vi "Capacitance Bridge.vi"(1 "Action":T4=enum."Identify", 2 "Parameters":variant) -> (6 "Output":variant, 7 "Stop":bool)   [LabVIEW 2020]
uses:
  Sub Controls/Instrument Actions.ctl
  Sub Controls/Public.ctl
  Sub Controls/Instrument Match.ctl
  Sub Controls/Factory Reset.ctl
  Sub Controls/Scan Output.ctl
  Sub Controls/Instrument IDN.ctl
  Sub Controls/User Event Command.ctl
panel:
  out "Firmware Warning":string="\nUPDATE Firmware!\nVersion must be ≥ AH2X0428"
  in  "Factory Reset":T1
  out "Average Time (mS)":u32
  in  "Read Frequency":bool
  out "Is AH2500?":bool
  out "Title":string="Capacitance Bridge"
  out "Frequency":dbl
  in  "Average Time":u32(slide)=4 max=15 step=1 scale=0.0..1.0
  in  "Return Dissapation":u8(slide) max=5 step=1 scale=0.0..5.0
  in  "VISA resource name":refnum<visa-resource-name>
  in  "Instruments":T2[](array[typedef])=[{"Model"="2500A", "Manufacturer"="ANDEEN-HAGERLING", "Term Character"="", "Wait Time (mS)"=0, "Wait for SRQ"=FALSE, "Type"="Capacitance Bridge"}, {"Model"="AH2700A", "Manufacturer"="ANDEEN-HAGERLING", "Term Character"="", "Wait Time (mS)"=0, "Wait for SRQ"=FALSE, "Type"="Capacitance Bridge"}]
  out "Model":string
  in  "Address":u16(ring)
  in  "Public":T3
  out "Measurement":dbl[](array[numeric]) format="%^.2e"
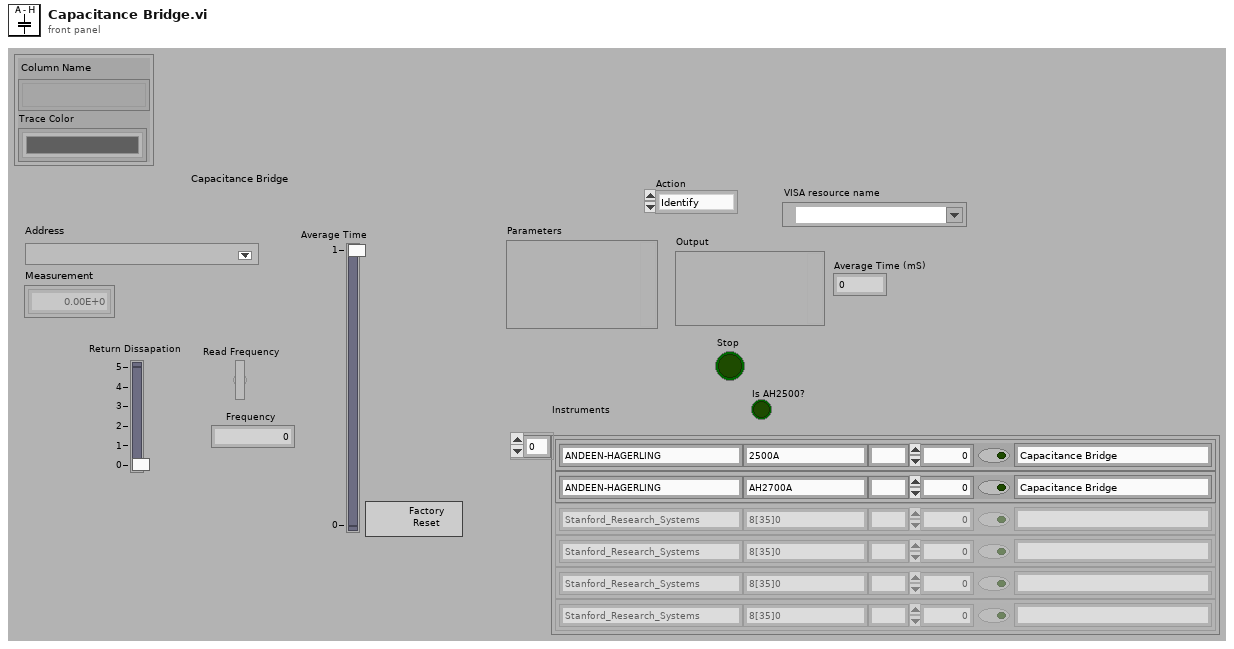
[diagram p1: front panel]
types:
  T1 = typedef "Factory Reset.ctl" = bool
  T2 = typedef "Instrument Match.ctl" = cluster{"Model":string, "Manufacturer":string, "Term Character":string, "Wait Time (mS)":u32, "Wait for SRQ":bool, "Type":string}
  T3 = typedef "Public.ctl" = cluster{"Column Name":string[], "Trace Color":u32[]}
  T4 = typedef "Instrument Actions.ctl" = enum16{"Scan", "Identify", "New", "Configure", "Initialize", "Test", "Read", "Close"}
  T5 = typedef "Scan Output.ctl" = cluster{"Manufacturer":string, "Model":string, "Info":string, "Revision":string, "error out":errorcluster}
  T6 = typedef "Instrument IDN.ctl" = cluster{"VISA Address":string, "Status":u16, "Manufacturer":string, "Model":string, "Info":string, "Info 2":string, "Misc Data":variant}
  T7 = typedef "User Event Command.ctl" = enum32{"Stop Config"}
  T8 = cluster{"VISA resource name":refnum<visa-resource-name>, string}
  T9 = typedef "Instrument Properties.ctl" = cluster{"Public":T3, "Private":T10}
  T10 = typedef "Private.ctl" = cluster{"Path":path, "VI Refnum":T11, "Name":string, "# of Values":i32, "Scale Factors":dbl[], "Display":T12[], "Offset":dbl[]}
  T11 = typedef "Instrument Ref.ctl" = refnum<vi>
  T12 = typedef "SystemCheckBox-resize.ctl" = bool
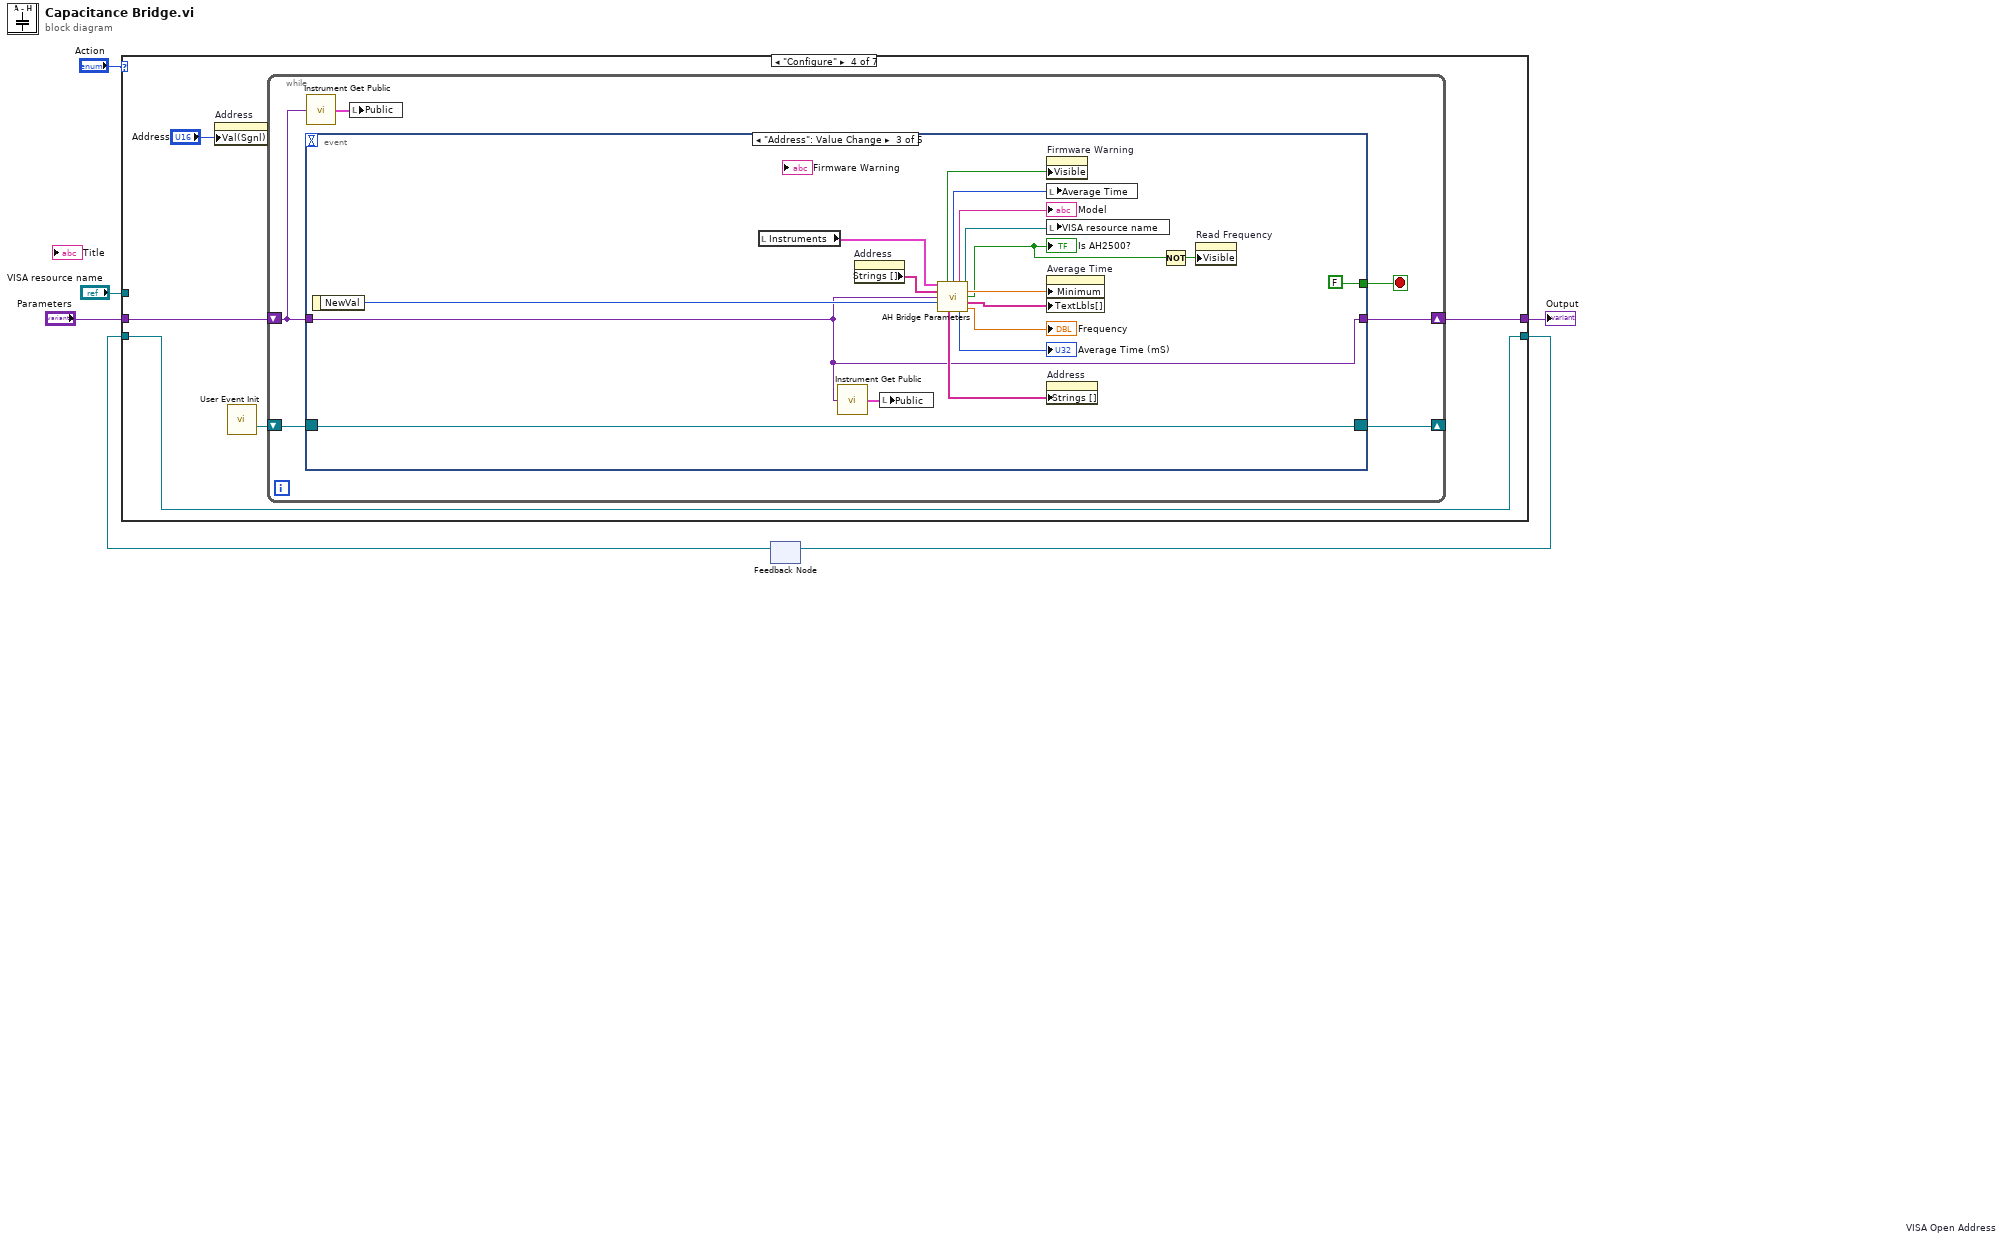
[diagram p0: block diagram]
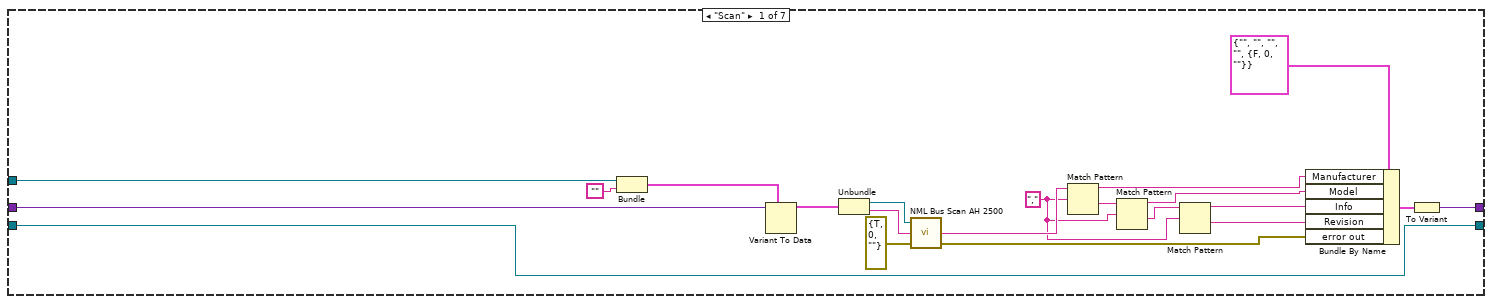
[diagram p2: hidden frame]
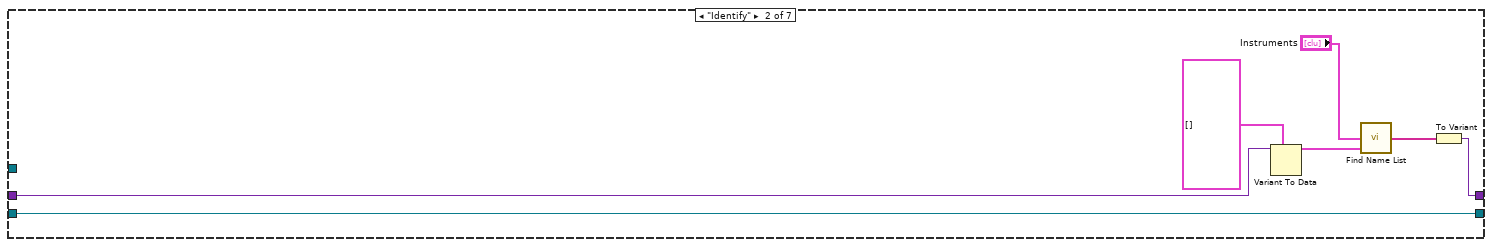
[diagram p3: hidden frame]
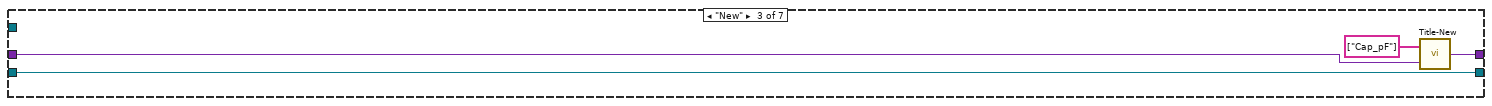
[diagram p4: hidden frame]
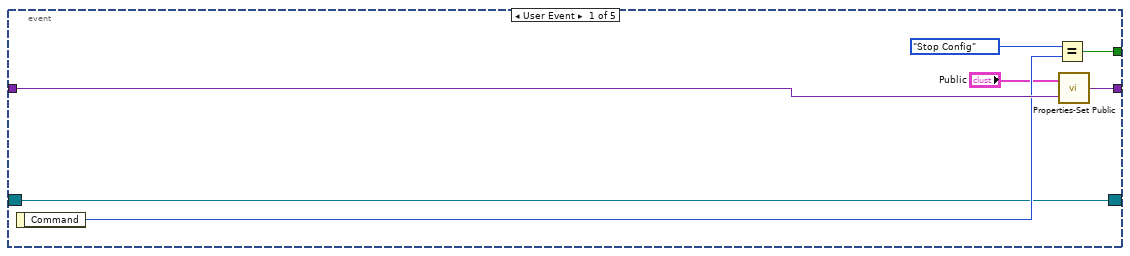
[diagram p5: hidden frame]
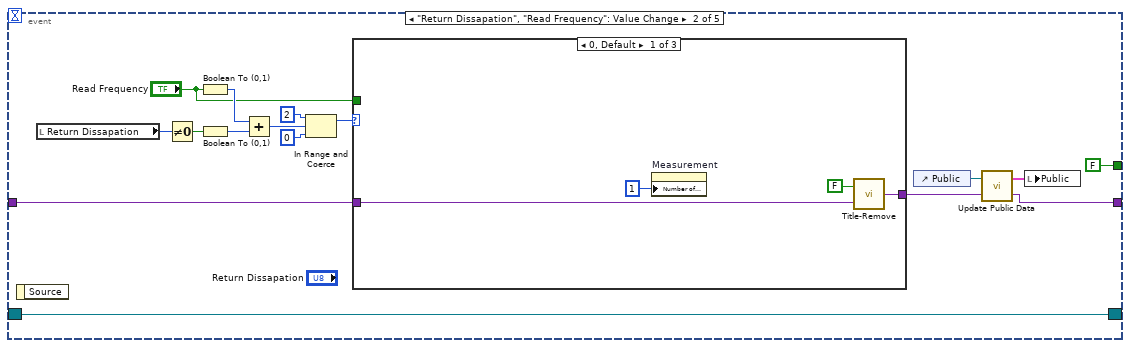
[diagram p6: hidden frame]
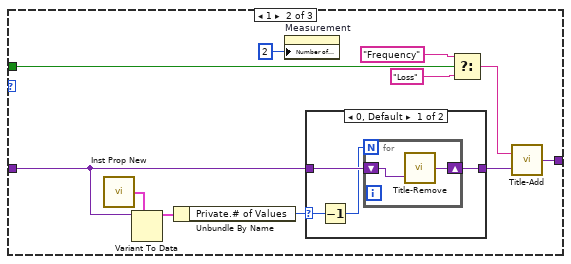
[diagram p7: hidden frame]
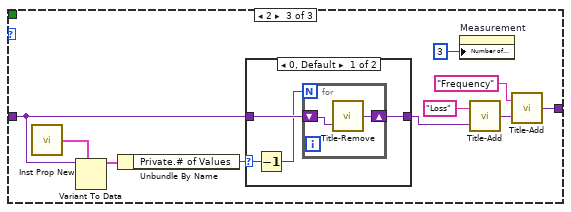
[diagram p9: hidden frame]
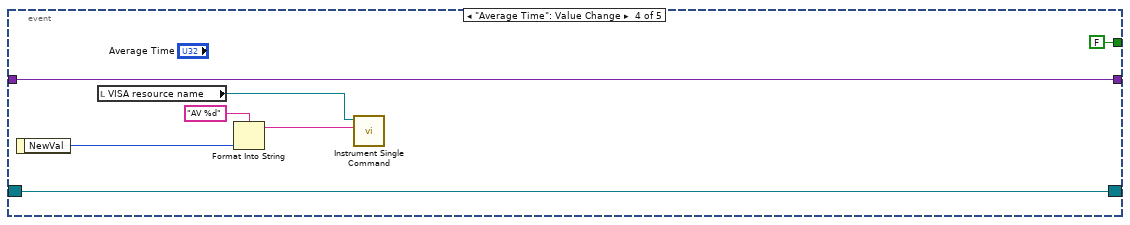
[diagram p11: hidden frame]
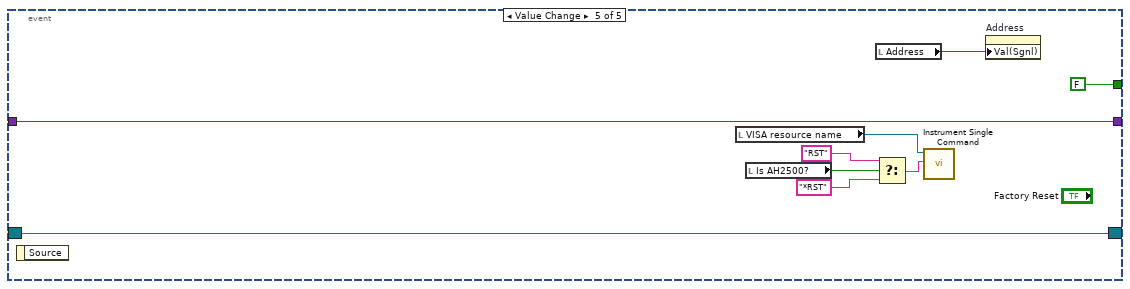
[diagram p12: hidden frame]
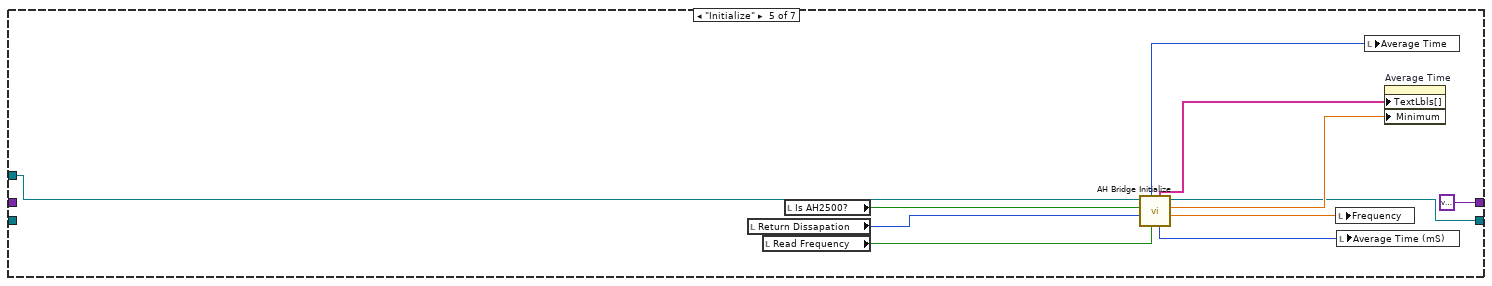
[diagram p13: hidden frame]
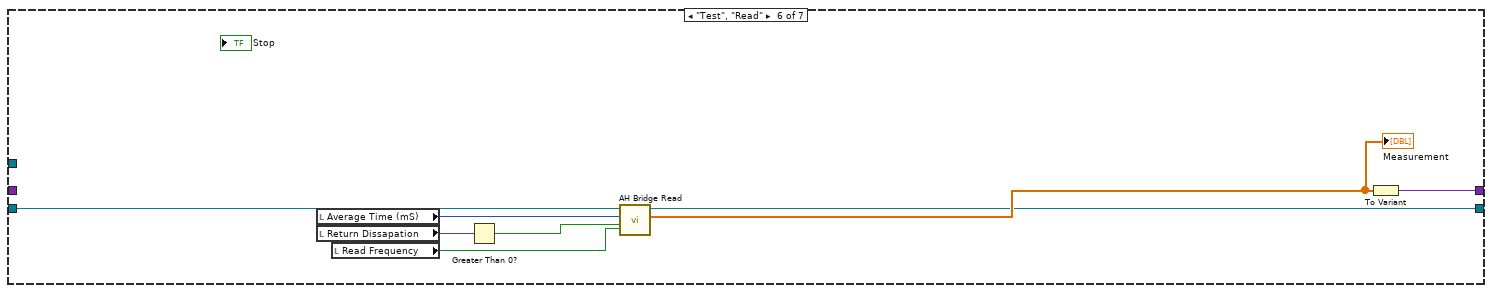
[diagram p14: hidden frame]
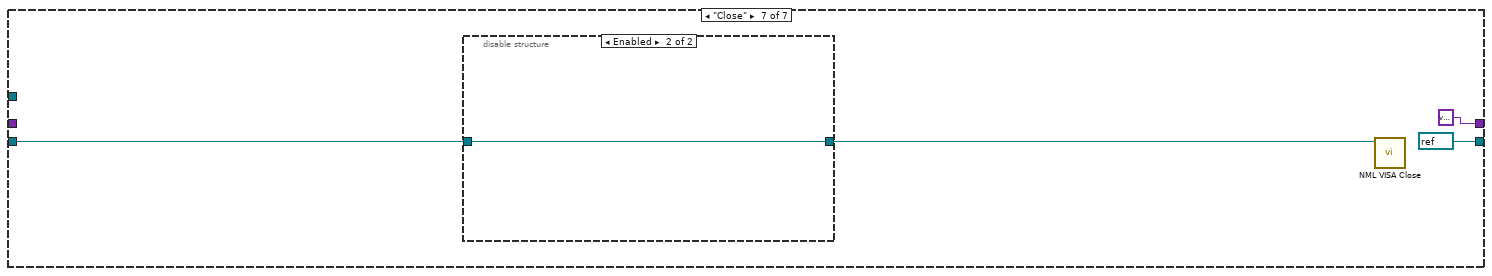
[diagram p15: hidden frame]
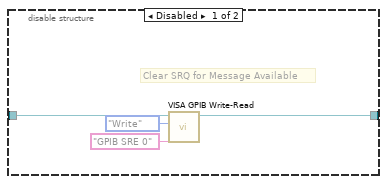
[diagram p16: hidden frame]
diagram:
  n1 = feedback #1 "VISA Open Address"() -> (w4:refnum<visa-resource-name>)  [unwired: 1 in]
  n2 = case shown="\"Configure\"" "Action" {
    tunnel: [w27 w34 w35 w39 w148 w161 refnum<visa-resource-name> refnum ("Open VISA Resource name")] -> w5
    tunnel: w4 -> [w27 w34 w35 w39 _ w157 w166]
    tunnel: "Parameters" -> [w22 w31 w37 w41 _ _ _]
    tunnel: [w26 w33 w36 w43 variant ("Variant") w164 variant ("Variant")] -> w2
    tunnel: "VISA resource name" -> [w25 _ _ _ w155 _ _]
    frame "Scan" {
      w14 = ","
      n3 = Bundle("VISA resource name"=w25, "") -> (w23:T8)  [unwired: 1 in]
      n4 = Variant To Data(type=w23, Variant=w22) -> (data=w21:T8)  [unwired: 1 in, 1 out]
      n5 = Unbundle(w21) -> ("VISA resource name"=w20:refnum<visa-resource-name>, w19:string)
      n6 = call "NML Bus Scan AH 2500.vi"("error in (no error)"=errorcluster {"status"=TRUE, "code"=0, "source"=""} ("error out"), "String Read In"=w19, "VISA Session"=w20) -> ("error out"=w7:errorcluster, "String Read Out"=w17:string)  [unwired: 1 out]
      n7 = Match Pattern(string=w17, regular expression=w14) -> (before substring=w9:string, after substring=w16:string)  [unwired: 1 in, 2 out]
      n8 = Match Pattern(string=w16, regular expression=w14) -> (before substring=w10:string, after substring=w15:string)  [unwired: 1 in, 2 out]
      n9 = Match Pattern(string=w15, regular expression=w14) -> (before substring=w11:string, after substring=w12:string)  [unwired: 1 in, 2 out]
      n10 = Bundle By Name(cluster=T5 {"Manufacturer"="", "Model"="", "Info"="", "Revision"="", "error out"={"status"=FALSE, "code"=0, "source"=""}} ("Scan Output"), "Manufacturer"=w9, "Model"=w10, "Info"=w11, "Revision"=w12, "error out"=w7) -> (w8:T5)
      n11 = To Variant(anything=w8) -> (Variant=w26:variant)
    }
    frame "Identify" {
      n12 = Variant To Data(type=T6[] [], Variant=w31) -> (data=w29:T6[])  [unwired: 1 in, 1 out]
      n13 = call "Find Name List.vi"("Bus Scan"=w29, "Instruments"="Instruments") -> ("Names"=w28:string[])  [unwired: 1 in]
      n14 = To Variant(anything=w28) -> (Variant=w33:variant)
    }
    frame "New" {
      n15 = call "Title-New.vi"("Parameters"=w37, "Array"=string[] ["Cap_pF"]) -> ("Instrument Prop"=w36:variant)
    }
    frame "Configure" {
      n16 = property on="Address" class="Ring (strict)"("Val(Sgnl)"="Address") -> ()  [unwired: 2 in, 2 out]
      n17 = call "User Event Init.vi"() -> ("Event Registration Refnum"=w42:refnum<event-registration>)  [unwired: 14 in, 1 out]
      n18 = while {
        shift-right: [w49] -> w43
        shift-left: w41 -> [w44]
        shift-right: [w46] -> _
        shift-left: w42 -> [w47]
        stop <- w48 stop-if-true
        n19 = event shown="[2] \"Address\": Value Change" {
          selector: w47 -> [w50 w71 w129 w130 w144]
          dyn-events: [w50 w71 w129 w130 w144] -> w46
          timeout: _ -> [_ _ _ _ _]
          tunnel: [w52 FALSE FALSE FALSE FALSE] -> w48
          tunnel: w44 -> [w55 w72 w115 w134 w145]
          tunnel: [w56 w69 w115 w134 w145] -> w49
          event User Event {
            n20 = event-data() -> ("Command"=w54:T7)  [unwired: 1 in]
            n21 = Equal?(x=User_Event_Command."Stop Config", y=w54) -> (x = y?=w52:bool)
            n22 = call "Properties-Set Public.vi"("Variant"=w55, "New Public"="Public") -> ("Variant 2"=w56:variant)
          }
          event "Return Dissapation", "Read Frequency": Value Change {
            n23 = event-data() -> ()  [unwired: 1 in, 1 out]
            n24 = local read "Return Dissapation"() -> (w58:u8)
            n25 = Not Equal To 0?(x=w58) -> (x != 0?=w65:bool)
            n26 = Boolean To (0,1)(Boolean="Read Frequency") -> (0, 1=w64:i16)
            n27 = Boolean To (0,1)(Boolean=w65) -> (0, 1=w63:i16)
            n28 = Add(x=w64, y=w63) -> (x+y=w61:i16)
            n29 = In Range and Coerce(upper limit=i16 2 ("x"), x=w61, lower limit=i16 0) -> (coerced(x)=w62:i16)  [unwired: 1 out]
            n30 = case shown="0, Default" w62 {
              tunnel: w72 -> [w75 w83 w96]
              tunnel: [w74 w87 w101] -> w70
              tunnel: "Read Frequency" -> [_ w77 _]
              frame 0, Default {
                n31 = property on="Measurement" class="Arr (strict)"("Number of Columns"=u32 1) -> ()  [unwired: 2 in, 2 out]
                n32 = call "Title-Remove.vi"("Parameters"=w75, "Remove First"=FALSE) -> ("Variant"=w74:variant)
              }
              frame 1 {
                n33 = call "Inst Prop New.vi"() -> ("Instrument Prop Out"=w84:T9)
                n34 = Variant To Data(type=w84, Variant=w83) -> (data=w85:T9)  [unwired: 1 in, 1 out]
                n35 = Unbundle By Name(w85) -> ("Private.# of Values"=w81:i32)
                n36 = property on="Measurement" class="Arr (strict)"("Number of Columns"=u32 2) -> ()  [unwired: 2 in, 2 out]
                n37 = case shown="0, Default" w81 {
                  selector: w81 -> [w88 _]
                  tunnel: w83 -> [w91 w94]
                  tunnel: [w90 w94] -> w82
                  frame 0, Default {
                    n38 = Decrement(x=w88) -> (x-1=w89:i32)
                    n39 = for {
                      N: w89 -> [_]
                      shift-right: [w93] -> w90
                      shift-left: w91 -> [w92]
                      n40 = call "Title-Remove.vi"("Parameters"=w92) -> ("Variant"=w93:variant)  [unwired: 1 in]
                    }
                  }
                  frame 1 {
                  }
                }
                n41 = Select(t="Frequency" ("String"), s=w77, f="Loss" ("String")) -> (s? t:f=w80:string)
                n42 = call "Title-Add.vi"("Parameters"=w82, "String"=w80) -> ("Variant"=w87:variant)
              }
              frame 2 {
                n43 = call "Inst Prop New.vi"() -> ("Instrument Prop Out"=w98:T9)
                n44 = Variant To Data(type=w98, Variant=w96) -> (data=w99:T9)  [unwired: 1 in, 1 out]
                n45 = Unbundle By Name(w99) -> ("Private.# of Values"=w95:i32)
                n46 = case shown="0, Default" w95 {
                  selector: w95 -> [w105 _]
                  tunnel: w96 -> [w108 w111]
                  tunnel: [w107 w111] -> w97
                  frame 0, Default {
                    n47 = Decrement(x=w105) -> (x-1=w106:i32)
                    n48 = for {
                      N: w106 -> [_]
                      shift-right: [w110] -> w107
                      shift-left: w108 -> [w109]
                      n49 = call "Title-Remove.vi"("Parameters"=w109) -> ("Variant"=w110:variant)  [unwired: 1 in]
                    }
                  }
                  frame 1 {
                  }
                }
                n50 = property on="Measurement" class="Arr (strict)"("Number of Columns"=u32 3) -> ()  [unwired: 2 in, 2 out]
                n51 = call "Title-Add.vi"("Parameters"=w97, "String"="Loss") -> ("Variant"=w102:variant)
                n52 = call "Title-Add.vi"("Parameters"=w102, "String"="Frequency") -> ("Variant"=w101:variant)
              }
            }
            n53 = control-ref of="Public"() -> (w67:refnum<vi>)
            n54 = call "Update Public Data.vi"("Variant In"=w70, "Public 2"=w67) -> ("Variant Out"=w69:variant, "Public"=w68:T3)
            n55 = local write "Public"(w68) -> ()
          }
          event "Address": Value Change {
            n56 = event-data() -> ("NewVal"=w120:u16)  [unwired: 1 in]
            n57 = local read "Instruments"() -> (w126:T2[])
            n58 = call "Instrument Get Public.vi"("Variant"=w115) -> ("Public"=w127:T3)
            n59 = property on="Address" class="Ring (strict)"() -> ("Strings []"=w125:string[])  [unwired: 2 in, 2 out]
            n60 = local write "Public"(w127) -> ()
            n61 = call "AH Bridge Parameters.vi"("Instruments"=w126, "NML Addresses"=w125, "Parameters"=w115, "Address"=w120) -> ("Show Firmware Warning"=w124:bool, "Setting"=w122:u32, "Model"=→"Model":string, "VISA Resource Name"=w114:refnum<visa-resource-name>, "Minimum"=w121:dbl, "Is AH 2500"=w112:bool, "Averaging Time"=w116:string[], "NML Addresses"=w123:string[], "Wait Time (mS)"=→"Average Time (mS)":u32, "Frequency"=→"Frequency":dbl)  [unwired: 1 in, 1 out]
            "Is AH2500?" <- w112
            n62 = property on="Firmware Warning" class="Str"("Visible"=w124) -> ()  [unwired: 2 in, 2 out]
            n63 = local write "Average Time"(w122) -> ()
            n64 = local write "VISA resource name"(w114) -> ()
            n65 = property on="Average Time" class="Slide (strict)"("Minimum"=w121, "TextLbls[]"=w116) -> ()  [unwired: 2 in, 2 out]
            n66 = property on="Address" class="Ring (strict)"("Strings []"=w123) -> ()  [unwired: 2 in, 2 out]
            n67 = Not(x=w112) -> (.not. x?=w113:bool)
            n68 = property on="Read Frequency" class="Bool (strict)"("Visible"=w113) -> ()  [unwired: 2 in, 2 out]
          }
          event "Average Time": Value Change {
            n69 = event-data() -> ("NewVal"=w136:u32)  [unwired: 1 in]
            n70 = local read "VISA resource name"() -> (w131:refnum<visa-resource-name>)
            n71 = Format Into String(format string="AV %d", w136) -> (resulting string=w132:string)  [unwired: 2 in, 1 out]
            n72 = call "Instrument Single Command.vi"("Reset Command"=w132, "VISA Name"=w131) -> ()  [unwired: 9 in, 1 out]
          }
          event Value Change {
            n73 = event-data() -> ()  [unwired: 1 in, 1 out]
            n74 = local read "VISA resource name"() -> (w137:refnum<visa-resource-name>)
            n75 = local read "Is AH2500?"() -> (w140:bool)
            n76 = local read "Address"() -> (w142:u16)
            n77 = Select(t="RST" ("Reset Command"), s=w140, f="*RST" ("Reset Command")) -> (s? t:f=w141:string)
            n78 = call "Instrument Single Command.vi"("Reset Command"=w141, "VISA Name"=w137) -> ()  [unwired: 9 in, 1 out]
            n79 = property on="Address" class="Ring (strict)"("Val(Sgnl)"=w142) -> ()  [unwired: 2 in, 2 out]
          }
        }
        n80 = call "Instrument Get Public.vi"("Variant"=w44) -> ("Public"=w45:T3)
        n81 = local write "Public"(w45) -> ()
      }
    }
    frame "Initialize" {
      n82 = local read "Return Dissapation"() -> (w150:u8)
      n83 = local read "Read Frequency"() -> (w151:bool)
      n84 = local read "Is AH2500?"() -> (w147:bool)
      n85 = call "AH Bridge Initialize.vi"("Read Frequency"=w151, "Return Dissapation"=w150, "Is AH2500?"=w147, "VISA Refnum in"=w155) -> ("Frequency"=w153:dbl, "Numeric"=w152:dbl, "VISA Refnum out"=w148:refnum<visa-resource-name>, "Wait Time (mS)"=w146:u32, "Averaging Time"=w154:string[], "Setting"=w149:u32)  [unwired: 2 in]
      n86 = local write "Frequency"(w153) -> ()
      n87 = local write "Average Time (mS)"(w146) -> ()
      n88 = local write "Average Time"(w149) -> ()
      n89 = property on="Average Time" class="Slide (strict)"("TextLbls[]"=w154, "Minimum"=w152) -> ()  [unwired: 2 in, 2 out]
    }
    frame "Test", "Read" {
      n90 = local read "Average Time (mS)"() -> (w158:u32)
      n91 = local read "Return Dissapation"() -> (w160:u8)
      n92 = local read "Read Frequency"() -> (w159:bool)
      n93 = Greater Than 0?(x=w160) -> (x > 0?=w163:bool)
      n94 = call "AH Bridge Read.vi"("Read Frequency"=w159, "Boolean"=w163, "Average Time (mS)"=w158, "Instrument Address"=w157) -> ("Measurement"=w162:dbl[], "dup Instrument Address"=w161:refnum<visa-resource-name>)  [unwired: 6 in]
      "Measurement" <- w162
      n95 = To Variant(anything=w162) -> (Variant=w164:variant)
    }
    frame "Close" {
      n96 = disable-structure shown="Enabled" {
        disable-tunnel: w166 -> [w172 w173]
        disable-tunnel: [w171 w173] -> w165
        frame Disabled {
          # "Clear SRQ for Message Available"
          n97 = call "VISA GPIB Write-Read.vi"("Command"="GPIB SRE 0", "Action"=enum16{"Write", "Read", "Write & Read"}."Write", "VISA resource name"=w172) -> ("dup VISA Session"=w171:refnum<visa-resource-name>)  [unwired: 5 in, 3 out]
        }
        frame Enabled {
        }
      }
      n98 = call "NML VISA Close.vi"("VISA resource name"=w165) -> ()  [unwired: 10 in, 1 out]
    }
  }
  "Output" <- w2
  n99 = feedback-in #1(w5) -> ()
